vi "Grabber Controller.vi"(8 "error in":errorcluster) -> ()   [LabVIEW 2017]
doc: "This VI executes continuously carrying out the current operation and responding to updates or new operations. It will often contain the timing or control code that is difficult to place directly in TeleOp. This VI generally opens all sensors and motors and isolates the rest of the robot code from knowing how the operations are carried out."
uses:
  <vilib>/Rock Robotics/WPI/Framework/Completion Status.ctl
  Grabber Setpoints.ctl
  Grabber Operations.ctl
  <vilib>/Rock Robotics/WPI/SafetyOutput/WPI_SafetyOutputConfigMenu.ctl
  <vilib>/Rock Robotics/SystemInterfaces/DIO/FPGA_DIOPWMChannel.ctl
  <vilib>/Rock Robotics/WPI/MotorControl/WPI_MotorControlOpen SPARK.vi
  <vilib>/Rock Robotics/Network Tables/NT Write Number.vi
panel:
  out "Setpoints":T1(graph)
  in  "Interactive Values":T2
  out "Current\nCmd":string
  in  "Buttons":cluster{"Execute Cmd":bool, "Abort Cmd":bool}
  out "Command Timing":cluster{"Start Time (ms)":u32, "Iterations":i32}
  out "Status":T4
  # "Tip: It may be helpful to observe inputs and sensor values.\nYou may also want to display tuning or debugging controls."
  # "Interactive Command: You may fill in the settings for a command\nand schedule it with the Execute button. You can observe and abort\nany command while fine tuning the code for the controller."
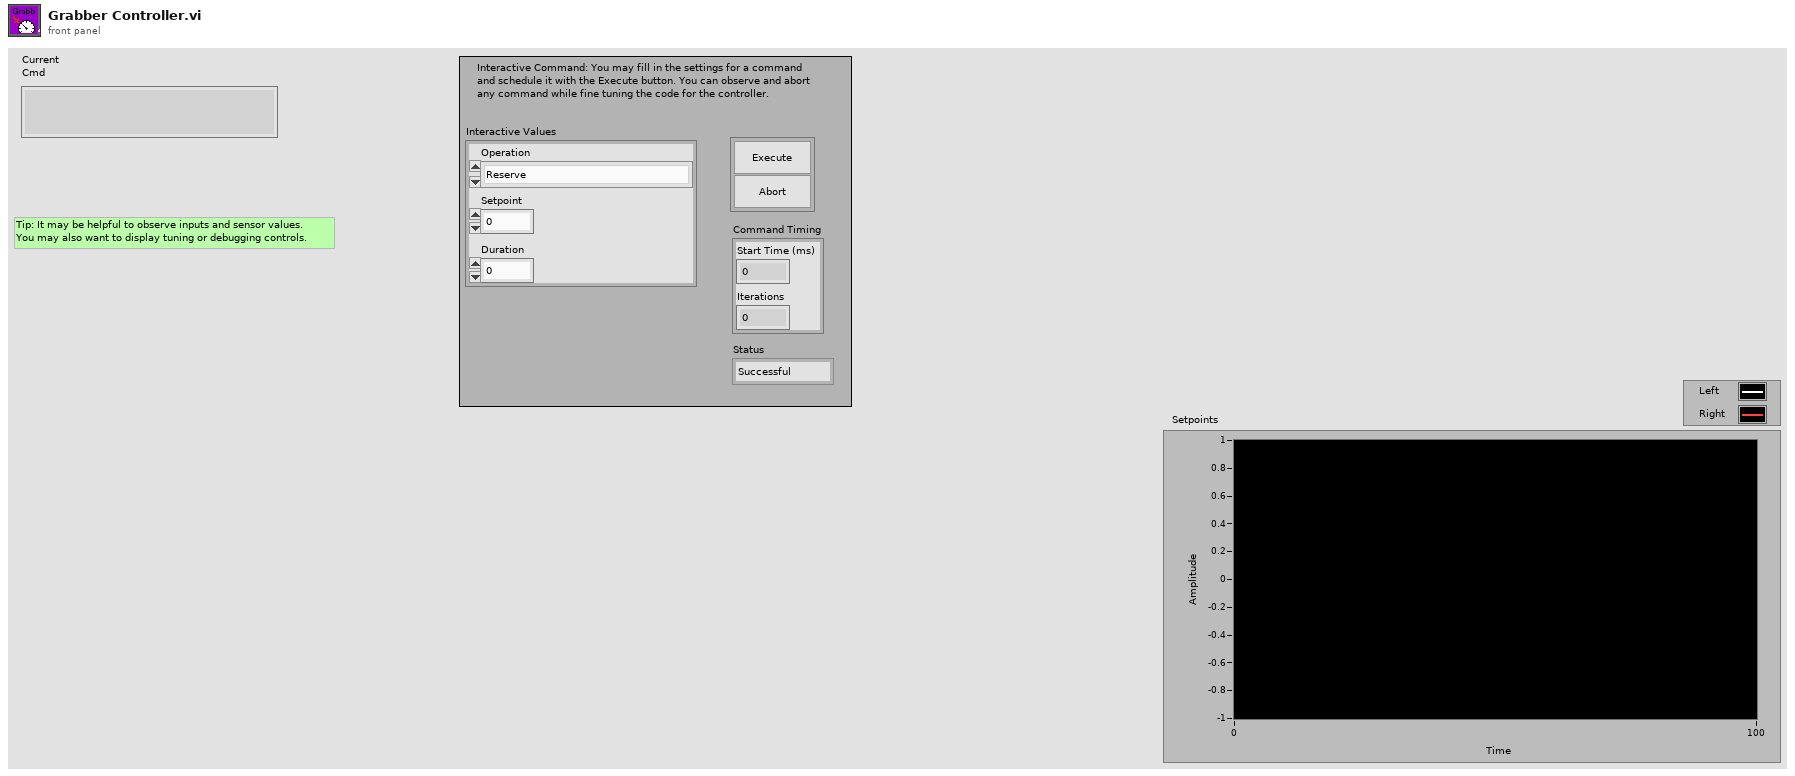
[diagram p1: front panel]
types:
  T1 = cluster{"Left Setpoint":dbl, "Right Setpoint":dbl}
  T2 = typedef "Grabber Setpoints.ctl" = cluster{"Operation":T3, "Setpoint":dbl, "Duration":dbl}
  T3 = typedef "Grabber Operations.ctl" = enum16{"Reserve", "Read Current", "Immediate", "Grab Power Cube", "Release Power Cube"}
  T4 = typedef "Completion Status.ctl" = enum16{"Successful", "Aborted", "Incomplete"}
  T5 = typedef "FPGA_DIOPWMChannel.ctl" = enum8{"PWM 0", "PWM 1", "PWM 2", "PWM 3", "PWM 4", "PWM 5", "PWM 6", "PWM 7", "PWM 8", "PWM 9", "PWM MXP 0", "PWM MXP 1", "PWM MXP 2", "PWM MXP 3", "PWM MXP 4", "PWM MXP 5", "PWM MXP 6", "PWM MXP 7", "PWM MXP 8", "PWM MXP 9", "Invalid"}
  T6 = typedef "WPI_SafetyOutputConfigMenu.ctl" = enum16{"Enable", "Disable"}
  T7 = typedef "WPI_MotorControlDeviceRef.ctl" = cluster{"DeviceStatus":errorcluster, "Type":T8, "PWM":cluster{"PWM Channel":T5, "DeadBand":T9}, "CAN":cluster{"Device Number":u8, "SetOutput VI Ref":variant, "GetOutput VI Ref":variant, "Enable VI Ref":variant, "Disable VI Ref":variant, "Data":variant}, "Invert":bool, "DIO PWM":cluster{"PWM \"Enable\" Channel":T5, "DIOChannel":T10, "PWM Rate":dbl}}
  T8 = typedef "WPI_MotorControlType.ctl" = enum16{"PWM", "CAN", "DIO PWM"}
  T9 = typedef "WPI_PWMDeadband.ctl" = cluster{"Name":string, "maxPositivePwm":i32, "minPositivePwm":i32, "centerPwm":i32, "maxNegativePwm":i32, "minNegativePwm":i32, "angularRange":u16}
  T10 = typedef "FPGA_DIOChannel.ctl" = enum8{"DIO 0", "DIO 1", "DIO 2", "DIO 3", "DIO 4", "DIO 5", "DIO 6", "DIO 7", "DIO 8", "DIO 9", "DIO MXP 0", "DIO MXP 1", "DIO MXP 2", "DIO MXP 3", "DIO MXP 4", "DIO MXP 5", "DIO MXP 6", "DIO MXP 7", "DIO MXP 8", "DIO MXP 9", "DIO MXP 10", "DIO MXP 11", "DIO MXP 12", "DIO MXP 13", "DIO MXP 14", "DIO MXP 15", "SPI Port CS1", "SPI Port CS2", "SPI Port CS3", "SPI Port MISO", "SPI Port MOSI", "Invalid"}
  T11 = typedef "Command Status Info.ctl" = cluster{"Name":string, "Status":T4, "notifier out":T12}
  T12 = typedef "Completion Notifier.ctl" = refnum<notifier>
  T13 = cluster{"Current Command":T2, "Command Timing":cluster{"Start Time (ms)":u32, "Iterations":i32}, "Command Arguments":cluster{"Command Info":T11, "Description":string, "Default Command":T2, "queue out":refnum<queue>, "Subsystem Name":string}}
  T14 = cluster{"Don't move motors while reserved":dbl, "Don't move motors while reserved":dbl}
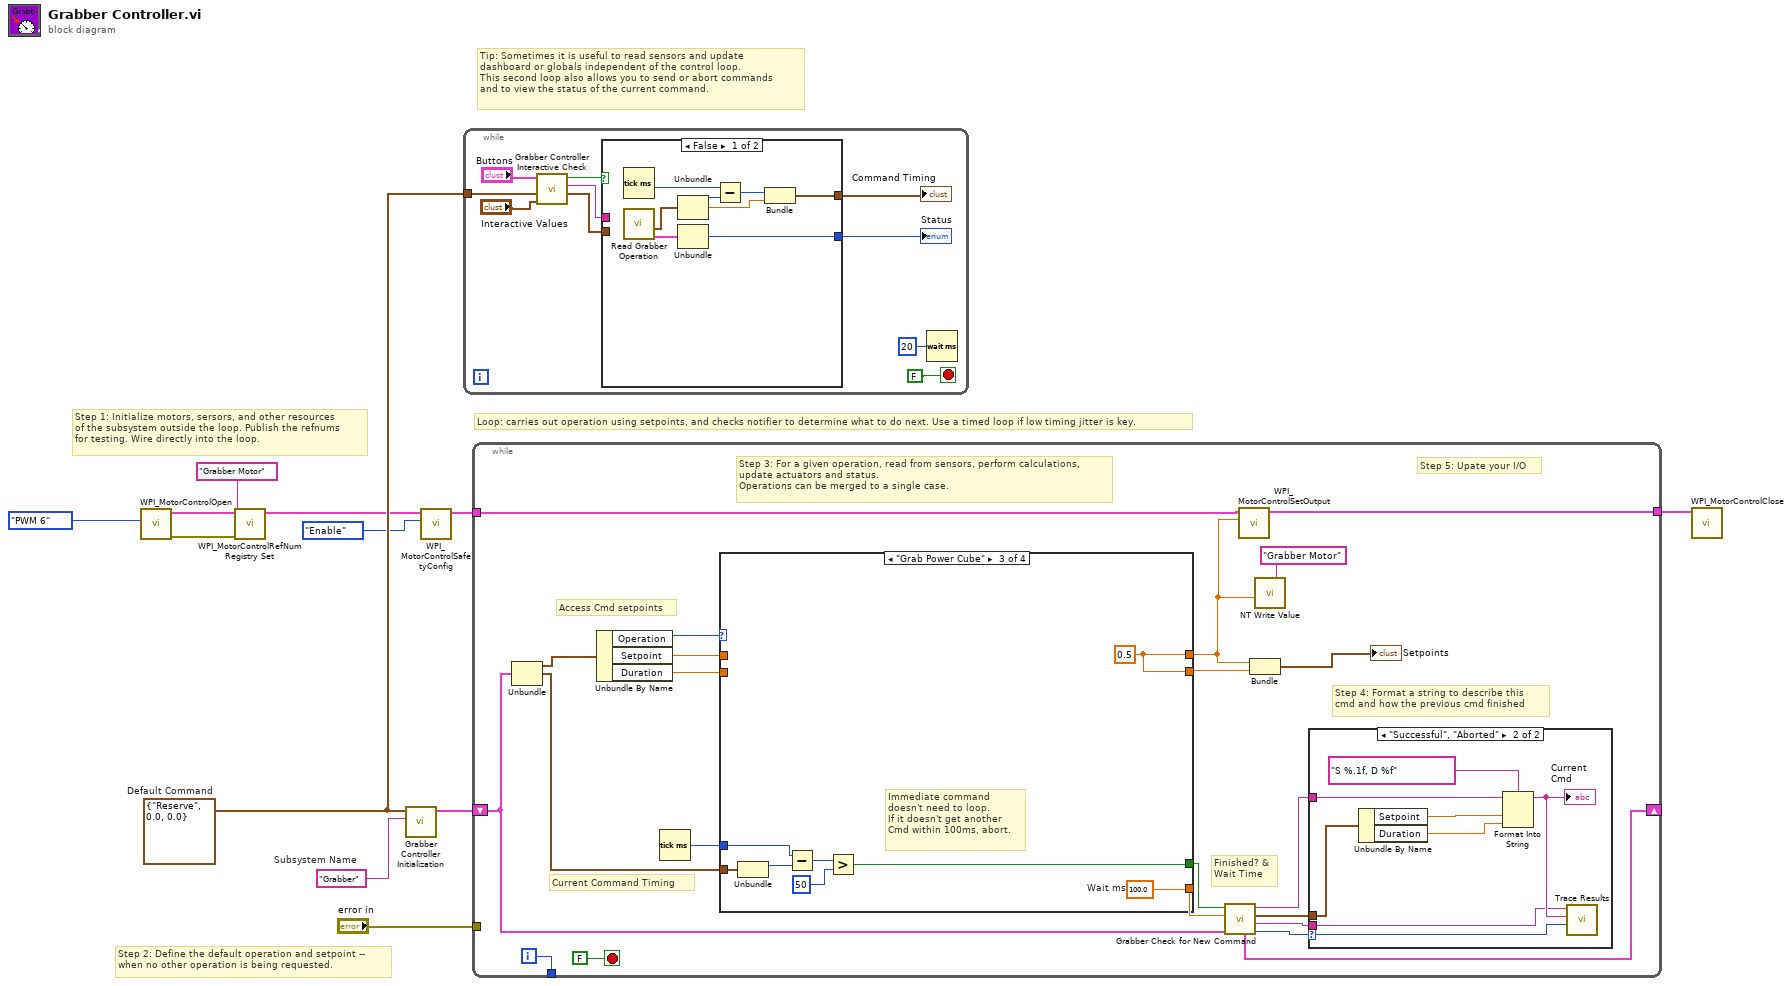
[diagram p0: block diagram]
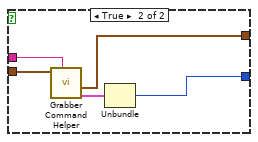
[diagram p2: hidden frame]
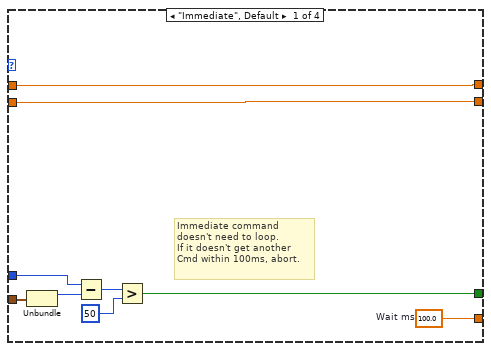
[diagram p4: hidden frame]
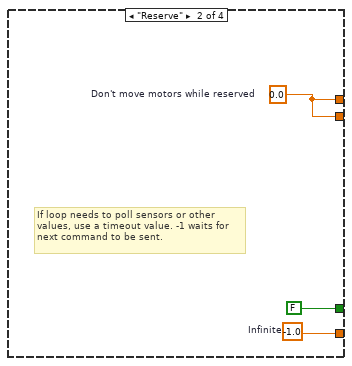
[diagram p5: hidden frame]
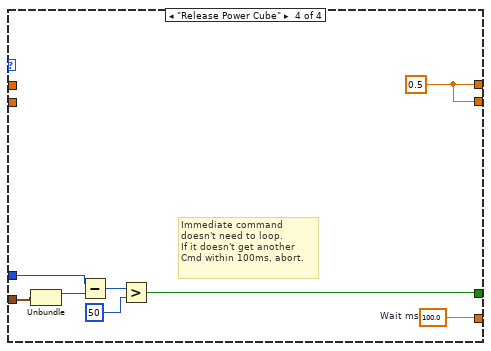
[diagram p6: hidden frame]
diagram:
  w9 = T2 {"Operation"=enum."Reserve", "Setpoint"=0.0, "Duration"=0.0}  # Default Command
  w10 = "Grabber"  # Subsystem Name
  # "Tip: Sometimes it is useful to read sensors and update\ndashboard or globals independent of the control loop.\nThis second loop also allows you to send or abort commands\nand to view the status of the current command."
  # "Step 2: Define the default operation and setpoint --\nwhen no other operation is being requested."
  # "Step 1: Initialize motors, sersors, and other resources\nof the subsystem outside the loop. Publish the refnums\nfor testing. Wire directly into the loop."
  # "Loop: carries out operation using setpoints, and checks notifier to determine what to do next. Use a timed loop if low timing jitter is key."
  n1 = call-poly <vilib>:"WPI_MotorControlOpen.vi"("PWM Channel"=FPGA_DIOPWMChannel."PWM 6") -> ("error out"=w8:errorcluster, "MotorControlDeviceRef"=w4:T7)  [unwired: 9 in]
  n2 = call <vilib>:"WPI_MotorControlRefNum Registry Set.vi"("error in (no error)"=w8, "refnum name"="Grabber Motor", "MotorControlDevRef"=w4) -> ("MotorControlDevRef"=w3:T7)  [unwired: 7 in, 1 out]
  n3 = call "Grabber Controller Initialization.vi"("Subsystem Name"=w10, "Default Command"=w9) -> ("Current Command"=w11:T13)  [unwired: 9 in]
  n4 = call <vilib>:"WPI_MotorControlSafetyConfig.vi"("mode"=WPI_SafetyOutputConfigMenu."Enable", "MotorControlDevRef"=w3) -> ("MotorControlDevRef"=w7:T7)  [unwired: 8 in, 1 out]
  n5 = while {
    tunnel: w9 -> [w19]
    stop <- FALSE stop-if-true
    n6 = call "Grabber Controller Interactive Check.vi"("Interactive Command in"="Interactive Values", "Default Command"=w19, "Buttons"="Buttons") -> ("Interactive Command out"=w16:T2, "Trace String"=w17:string, "Schedule"=w18:bool)  [unwired: 6 in]
    n7 = case shown="False" w18 {
      tunnel: [w30 w35] -> w15
      tunnel: w16 -> [_ w33]
      tunnel: [w26 w31] -> w14
      tunnel: w17 -> [_ w34]
      frame False {
        n8 = Tick Count (ms)() -> (millisecond timer value=w25:u32)
        n9 = call "Read Grabber Operation.vi"() -> ("Command Info"=w23:T11, "SubSystem Data"=w24:T2)  [unwired: 9 in, 1 out]
        n10 = Unbundle(w24) -> ("Operation"=w29:T3, "Setpoint"=w27:dbl)  [unwired: 1 out]
        n11 = Unbundle(w23) -> ("Status"=w30:T4)  [unwired: 2 out]
        n12 = Subtract(x=w25, y=w29) -> (x-y=w28:u32)
        n13 = Bundle(w28, "Setpoint"=w27) -> (w26:cluster{u32, "Setpoint":dbl})  [unwired: 1 in]
      }
      frame True {
        n14 = call "Grabber Command Helper.vi"("Description"=w34, "SubSystem Data"=w33) -> ("Command Info Out"=w32:T11, "Command Timing"=w31:cluster{"Start Time (ms)":u32, "Iterations":i32})  [unwired: 7 in, 1 out]
        n15 = Unbundle(w32) -> ("Status"=w35:T4)  [unwired: 2 out]
      }
    }
    "Status" <- w15
    "Command Timing" <- w14
    n16 = Wait (ms)(milliseconds to wait=u32 20) -> ()  [unwired: 1 out]
  }
  n17 = while {
    shift-right: [w49] -> _
    shift-left: w11 -> [w42]
    tunnel: [w56] -> _
    tunnel: "error in" -> [_]
    tunnel: w7 -> [w41]
    tunnel: [w36] -> w1
    i -> [w56]
    stop <- FALSE stop-if-true
    # "Step 5: Upate your I/O"
    # "Step 4: Format a string to describe this\ncmd and how the previous cmd finished"
    # "Current Command Timing"
    # "Access Cmd setpoints"
    # "Finished? &\nWait Time"
    # "Step 3: For a given operation, read from sensors, perform calculations,\nupdate actuators and status.\nOperations can be merged to a single case."
    n18 = Unbundle(w42) -> ("Current Command"=w55:T2, "Command Timing"=w51:cluster{"Start Time (ms)":u32, "Iterations":i32})  [unwired: 1 out]
    n19 = Unbundle By Name(w55) -> ("Operation"=w54:T3, "Setpoint"=w53:dbl, "Duration"=w50:dbl)
    n20 = Tick Count (ms)() -> (millisecond timer value=w52:u32)
    n21 = case shown="\"Grab Power Cube\"" w54 {
      tunnel: [w74 w77 w79 w87] -> w47
      tunnel: [w68 FALSE ("ignore previous (F)") w80 w88] -> w48
      tunnel: w51 -> [w70 _ w83 w90]
      tunnel: w53 -> [w67 _ _ _]
      tunnel: w52 -> [w69 _ w82 w91]
      tunnel: w50 -> [w66 _ _ _]
      tunnel: [w67 w75 w78 w86] -> w38
      tunnel: [w66 w75 w78 w86] -> w39
      frame "Immediate", Default {
        w74 = 100.0  # Wait ms
        # "Immediate command\ndoesn't need to loop.\nIf it doesn't get another\nCmd within 100ms, abort."
        n22 = Unbundle(w70) -> ("Start Time (ms)"=w73:u32)  [unwired: 1 out]
        n23 = Subtract(x=w69, y=w73) -> (x-y=w72:u32)
        n24 = Greater?(x=w72, y=u8 50 ("Left Motor")) -> (0:w68:bool)
      }
      frame "Reserve" {
        w75 = 0.0  # Don't move motors while reserved
        w77 = -1.0  # Infinite
        # "If loop needs to poll sensors or other\nvalues, use a timeout value. -1 waits for\nnext command to be sent."
      }
      frame "Grab Power Cube" {
        w78 = 0.5 ("Don't move motors while reserved")
        w79 = 100.0  # Wait ms
        # "Immediate command\ndoesn't need to loop.\nIf it doesn't get another\nCmd within 100ms, abort."
        n25 = Unbundle(w83) -> ("Start Time (ms)"=w81:u32)  [unwired: 1 out]
        n26 = Subtract(x=w82, y=w81) -> (x-y=w85:u32)
        n27 = Greater?(x=w85, y=u8 50 ("Left Motor")) -> (0:w80:bool)
      }
      frame "Release Power Cube" {
        w86 = 0.5 ("Don't move motors while reserved")
        w87 = 100.0  # Wait ms
        # "Immediate command\ndoesn't need to loop.\nIf it doesn't get another\nCmd within 100ms, abort."
        n28 = Unbundle(w90) -> ("Start Time (ms)"=w89:u32)  [unwired: 1 out]
        n29 = Subtract(x=w91, y=w89) -> (x-y=w93:u32)
        n30 = Greater?(x=w93, y=u8 50 ("Left Motor")) -> (0:w88:bool)
      }
    }
    n31 = call "Grabber Check for New Command.vi"("Current Command"=w42, "Wait time (ms)"=w47, "Finished?"=w48) -> ("Completion"=w43:T4, "Subsystem Name"=w44:string, "Current Command"=w45:T2, "Initial Trace String"=w46:string, "NextCommand"=w49:T13)  [unwired: 4 in]
    n32 = call <vilib>:"WPI_MotorControlSetOutput.vi"("Output"=w38, "MotorControlDevRef"=w41) -> ("MotorControlDevRef"=w36:T7)  [unwired: 7 in, 2 out]
    n33 = Bundle("Don't move motors while reserved"=w38, "Don't move motors while reserved"=w39) -> (→"Setpoints":T14)  [unwired: 1 in]
    n34 = call-poly <vilib>:"NT Write Value.vi"("Numeric"=w38, "Name"="Grabber Motor") -> ()  [unwired: 9 in, 1 out]
    n35 = case shown="\"Successful\", \"Aborted\"" w43 {
      selector: w43 -> [_ w65]
      tunnel: w46 -> [_ w61]
      tunnel: w45 -> [_ w62]
      tunnel: w44 -> [_ w58]
      frame "Incomplete", Default {
        # "Continuing current command"
      }
      frame "Successful", "Aborted" {
        # "Report and setup for next command"
        n36 = Unbundle By Name(w62) -> ("Setpoint"=w64:dbl, "Duration"=w59:dbl)
        n37 = Format Into String(format string="S %.1f, D %f", initial string=w61, w64, w59) -> (resulting string=w60:string)  [unwired: 1 in, 1 out]
        "Current\nCmd" <- w60
        n38 = call <vilib>:"Trace Results.vi"("Status of previous command"=w65, "Description"=w60, "Subsystem"=w58) -> ()  [unwired: 9 in]
      }
    }
  }
  n39 = call <vilib>:"WPI_MotorControlClose.vi"("MotorControlDevRef"=w1) -> ()  [unwired: 10 in, 1 out]
